vi "USB Memory Get Catalog All.vi"(8 "error in (no error)":errorcluster {"code" format="%.0x"}, 9 "ListOfFilesBufferSize":i32=256, 11 "instrument handle":refnum<k15>) -> (0 "error out":errorcluster {"code" format="%.0x"}, 1 "MemoryFree":i64, 2 "MemoryUsed":i64, 3 "instrument handle out":refnum<k15>, 4 "ListOfFiles":string)   [LabVIEW 2020, in "Keysight DAQ970.lvlib"]
doc: "Returns the memory usage information (used and free space) and list of files (for each file : name, type and size) in the memory subsystem."
uses:
  Keysight DAQ970.lvlib
  KtDAQ970.dll
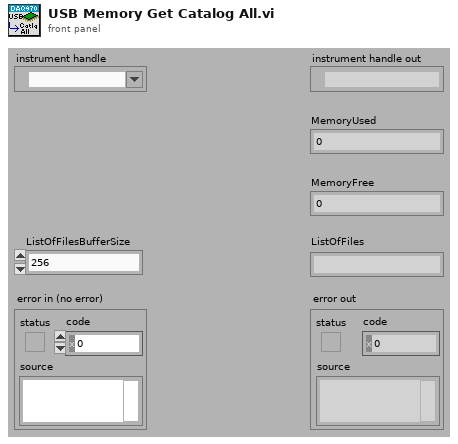
[diagram p1: front panel]
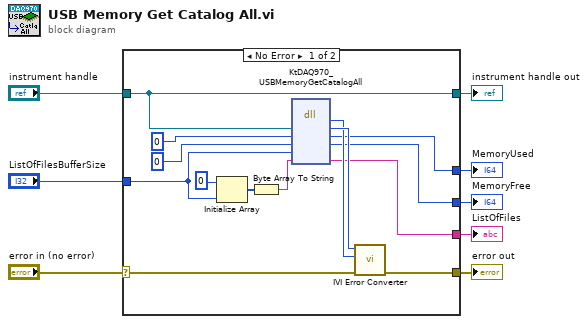
[diagram p0: block diagram]
diagram:
  n1 = case shown="No Error" "error in (no error)" {
    selector: "error in (no error)" -> [w20 w24]
    tunnel: [w19 w24] -> w8
    tunnel: "instrument handle" -> [w10 w23]
    tunnel: [w17 _] -> w5
    tunnel: [w15 _] -> w4
    tunnel: "ListOfFilesBufferSize" -> [w9 _]
    tunnel: [w11 _] -> w2
    tunnel: [w10 w23] -> w1
    frame No Error {
      n2 = Initialize Array(u8 0 ("element"), w9) -> (w13:u8[])
      n3 = Byte Array To String(unsigned byte array=w13) -> (string=w14:string)
      n4 = dll-call lib="KtDAQ970**.dll" fn="KtDAQ970_USBMemoryGetCatalogAll"("Vi"=w10, "MemoryUsed"=i64 0, "MemoryFree"=i64 0, "ListOfFilesBufferSize"=w9, "ListOfFiles"=w14) -> (w21:i32, "Vi"=w22:u32, "MemoryUsed"=w17:i64, "MemoryFree"=w15:i64, "ListOfFiles"=w11:string)  [unwired: 4 in, 2 out]
      n5 = call "IVI Error Converter.vi"("error in (no error)"=w20, "IVI error code (0)"=w21, "instrument handle"=w22) -> ("error out"=w19:errorcluster)  [unwired: 7 in, 1 out]
    }
    frame Error {
    }
  }
  "error out" <- w8
  "instrument handle out" <- w1
  "MemoryUsed" <- w5
  "MemoryFree" <- w4
  "ListOfFiles" <- w2
